vi "pp_sessionList_isValid.vi"(0 "Trial Types":T1(array[cluster]) {"Stim P2" min=0.0; "Trial Weight" step=1; "Stim P1" min=0.0; "Stim Dur (s)" min=0.0; "Trial Code" min=1 step=1}, 5 "Total Trials":i32=60 min=2 step=2, 7 "Trial Replication Factor":i32, 9 "Session List":i32[](array[numeric])) -> (4 "Session List Valid?":bool=TRUE)   [LabVIEW 2013]
uses:
  labolabo/array/impl/ArrayRemove_I.vi
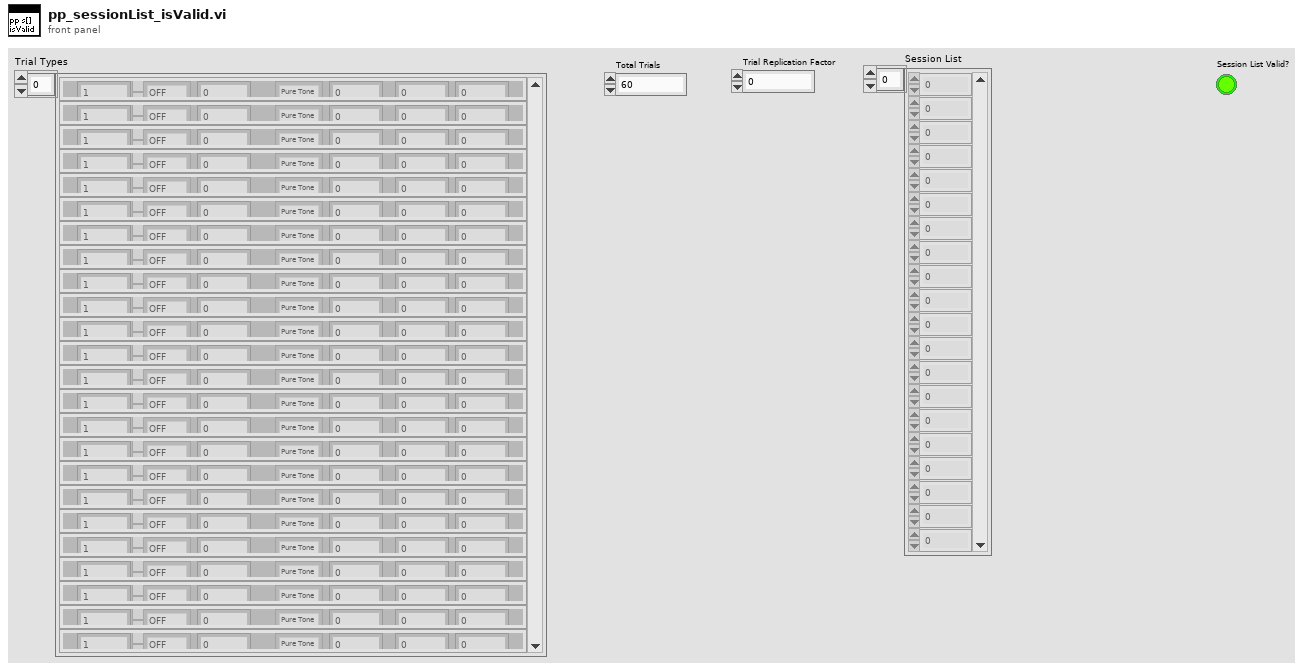
[diagram p1: front panel]
types:
  T1 = cluster{"Trial Code":u16, "Trial Type":enum16{"OFF", "GO", "NOGO", "TEST"}, "Trial Weight":u32, "Stim Type":enum16{"Pure Tone", "FM Sweep"}, "Stim Dur (s)":dbl, "Stim P1":dbl, "Stim P2":dbl}[]
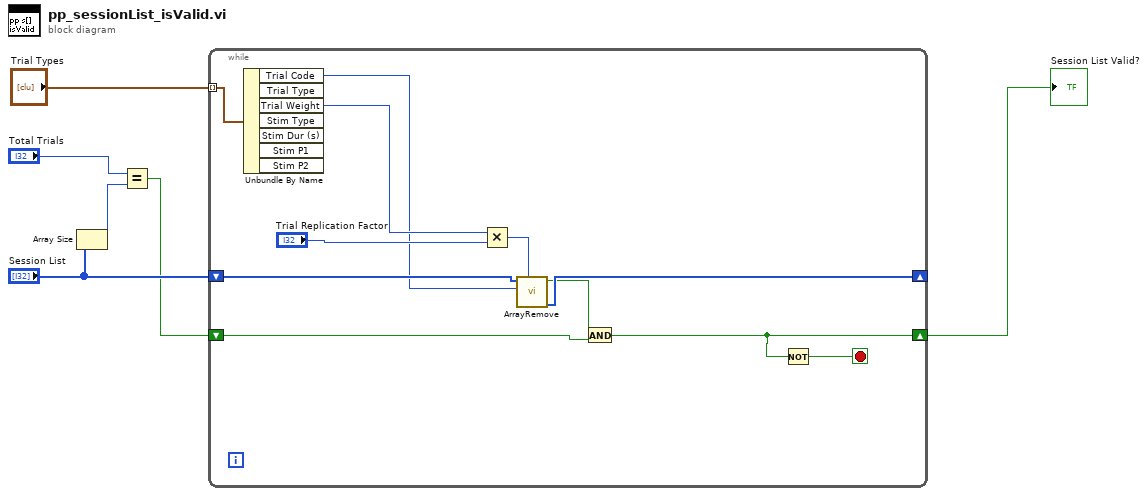
[diagram p0: block diagram]
diagram:
  n1 = Array Size(array="Session List") -> (size(s)=w6:i32)
  n2 = Equal?(x="Total Trials", y=w6) -> (x = y?=w2:bool)
  n3 = while {
    tunnel: "Trial Types" -> [w17] mode=indexing
    shift-right: [w15] -> _
    shift-left: "Session List" -> [w16]
    shift-right: [w8] -> w1
    shift-left: w2 -> [w13]
    stop <- w7 stop-if-true
    n4 = Unbundle By Name(w17) -> ("Trial Code"=w9:u16, "Trial Weight"=w12:u32)  [unwired: 5 out]
    n5 = Multiply(x=w12, y="Trial Replication Factor") -> (x*y=w10:u32)
    n6 = call-poly "ArrayRemove.vi"("N"=w10, "To Remove"=w9, "1D Array In"=w16) -> ("1D Array Out"=w15:i32[], "Removed All"=w14:bool)  [unwired: 7 in]
    n7 = And(x=w14, y=w13) -> (x .and. y?=w8:bool)
    n8 = Not(x=w8) -> (.not. x?=w7:bool)
  }
  "Session List Valid?" <- w1
